vi "ELVIS III v1.0 Read AI.vi"(7 "Scale Constants Array":T1, 8 "error in (no error)":errorcluster, 10 "Channel List":T5, 11 "myRIO Ref In":T3) -> (0 "error out":errorcluster, 2 "dbl Scaled Value List":dbl[](array[numeric]), 3 "myRIO Ref Out":T3)   [LabVIEW 2021]
uses:
  <vilib>/myRIO/Common/Instrument Driver Framework/myRIO v1.0/AI/typedefs/AI Channels List.ctl
  <vilib>/myRIO/Common/Instrument Driver Framework/myRIO v1.0/AI/typedefs/AI Channels Enum.ctl
  <vilib>/myRIO/Common/Instrument Driver Framework/Utilities/typedefs/myRIO v1.0 Reference.ctl
  <vilib>/myRIO/Common/Instrument Driver Framework/Utilities/typedefs/Generic FPGA Reference.ctl
  <vilib>/myRIO/Common/Instrument Driver Framework/Utilities/typedefs/Analog Scaling Constants List.ctl
  <vilib>/myRIO/Common/Instrument Driver Framework/Utilities/typedefs/Analog Scaling Constants.ctl
  <vilib>/myRIO/Common/Instrument Driver Framework/ELVIS III v1.0/AI/typedefs/ELVIS III AI Channels FPGA Reference.ctl
  <vilib>/rvi/errors/niLvFpgaAdjustHostInterfaceError.vi
  <vilib>/rvi/interface/nirviReadWriteControl/nirviReadWriteControl.xnode
  <vilib>/rvi/interface/Simulation/niFpgaSimulationCallBeginRW.vi
  NiFpgaLv.dll
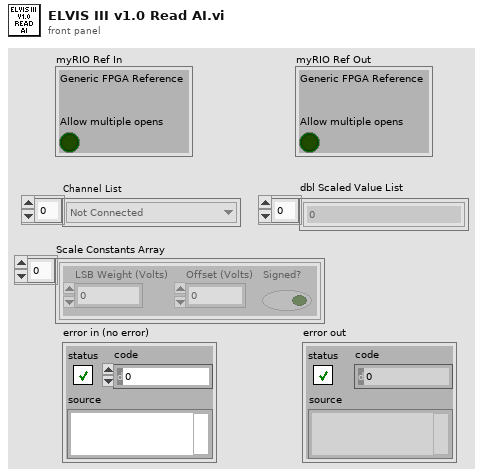
[diagram p1: front panel]
types:
  T1 = typedef "Analog Scaling Constants List.ctl" = T2[]
  T2 = typedef "Analog Scaling Constants.ctl" = cluster{"LSB Weight (Volts)":dbl, "Offset (Volts)":dbl, "Signed?":bool}
  T3 = typedef "myRIO v1.0 Reference.ctl" = cluster{"Generic FPGA Reference":T4, "Allow multiple opens":bool}
  T4 = typedef "Generic FPGA Reference.ctl" = refnum<k20>
  T5 = typedef "AI Channels List.ctl" = T6[]
  T6 = typedef "AI Channels Enum.ctl" = enum16{"Not Connected", "AudioIn/Left", "AudioIn/Right", "C/AI0", "C/AI1", "A/AI0", "A/AI1", "A/AI2", "A/AI3", "A/AI4", "A/AI5", "A/AI6", "A/AI7", "B/AI0", "B/AI1", "B/AI2", "B/AI3", "B/AI4", "B/AI5", "B/AI6", "B/AI7", "AI/AI0", "AI/AI1", "AI/AI2", "AI/AI3", "A/AI0 (DIFF)", "A/AI1 (DIFF)", "A/AI2 (DIFF)", "A/AI3 (DIFF)", "B/AI0 (DIFF)", "B/AI1 (DIFF)", "B/AI2 (DIFF)", "B/AI3 (DIFF)"}
  T7 = typedef "ELVIS III AI Channels FPGA Reference.ctl" = refnum<k20>
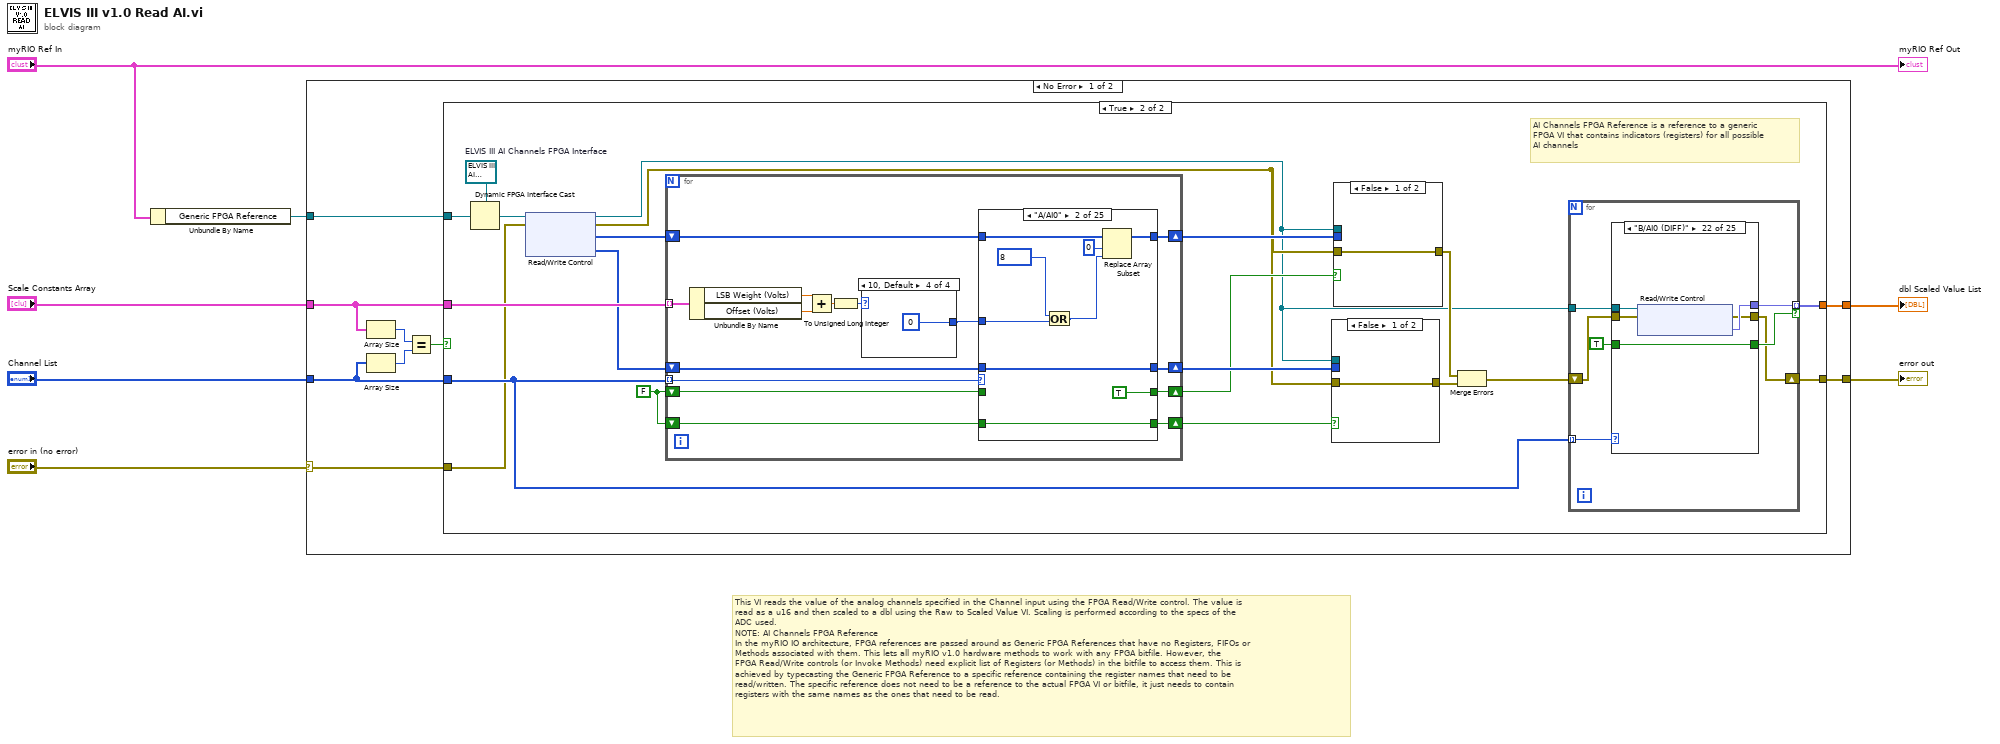
[diagram p0: block diagram]
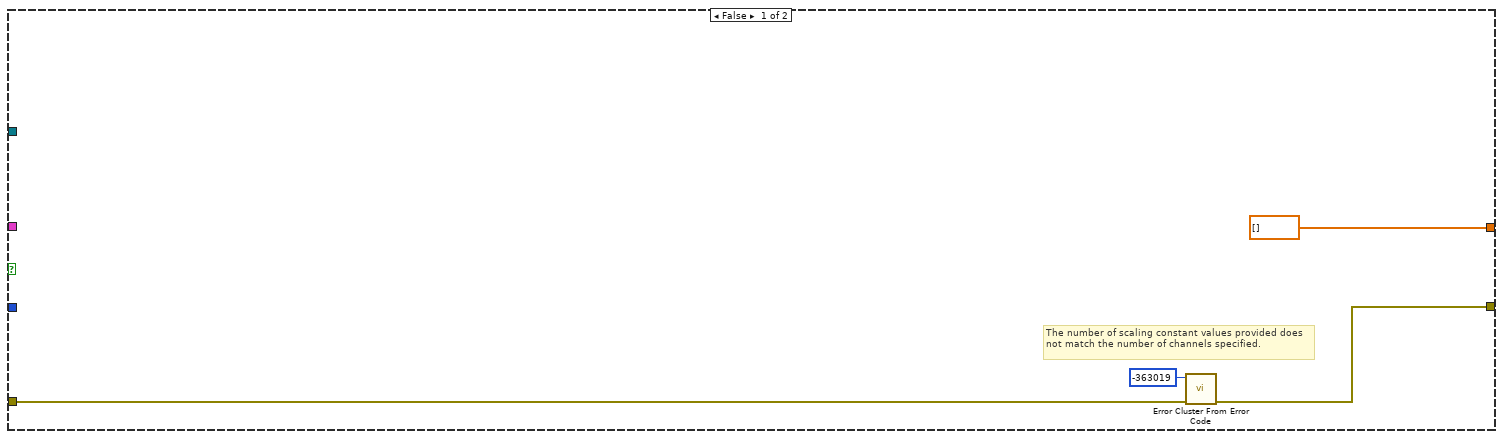
[diagram p2: hidden frame]
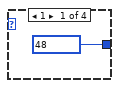
[diagram p3: hidden frame]
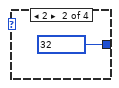
[diagram p4: hidden frame]
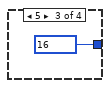
[diagram p5: hidden frame]
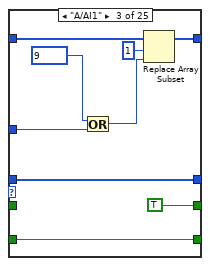
[diagram p7: hidden frame]
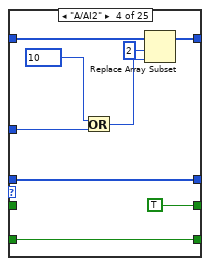
[diagram p8: hidden frame]
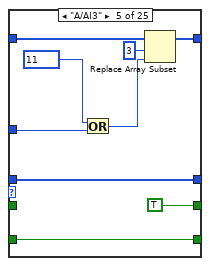
[diagram p9: hidden frame]
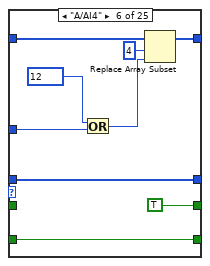
[diagram p10: hidden frame]
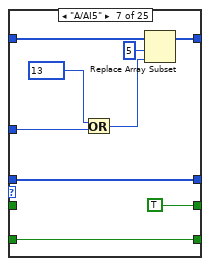
[diagram p11: hidden frame]
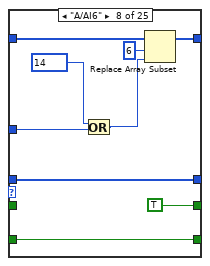
[diagram p12: hidden frame]
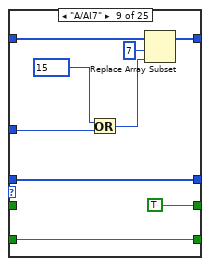
[diagram p13: hidden frame]
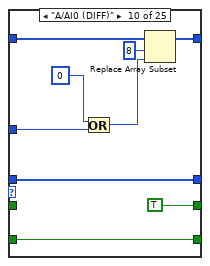
[diagram p14: hidden frame]
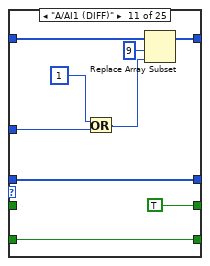
[diagram p15: hidden frame]
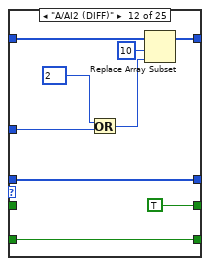
[diagram p16: hidden frame]
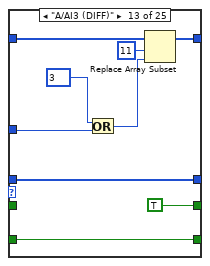
[diagram p17: hidden frame]
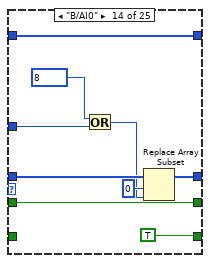
[diagram p18: hidden frame]
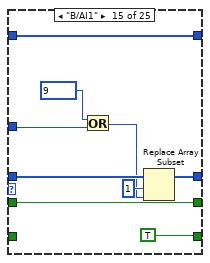
[diagram p19: hidden frame]
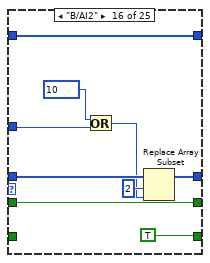
[diagram p20: hidden frame]
diagram:
  # "This VI reads the value of the analog channels specified in the Channel input using the FPGA Read/Write control. The value is \nread as a u16 and then scaled to a dbl using the Raw to Scaled Value VI. Scaling is performed according to the specs of the \nADC used.\nNOTE: AI Channels FPGA Reference\nIn the myRIO IO architecture, FPGA references are passed around as Generic FPGA References that have no Registers, FIFOs or\nMethods associated with them. This lets all myRIO v1.0 hardware methods to work with any FPGA bitfile. However, the \nFPGA Read/Write controls (or Invoke Methods) need explicit list of Registers (or Methods) in the bitfile to access them. This is \nachieved by typecasting the Generic FPGA Reference to a specific reference containing the register names that need to be \nread/written. The specific reference does not need to be a reference to the actual FPGA VI or bitfile, it just needs to contain \nregisters with the same names as the ones that need to be read."
  n1 = Unbundle By Name("myRIO Ref In") -> ("Generic FPGA Reference"=w3:T4)
  n2 = case shown="No Error" "error in (no error)" {
    selector: "error in (no error)" -> [w9 w421]
    tunnel: w3 -> [w16 _]
    tunnel: [w15 w421] -> w7
    tunnel: "Channel List" -> [w13 _]
    tunnel: "Scale Constants Array" -> [w14 _]
    tunnel: [w8 dbl[] []] -> w1
    frame No Error {
      n3 = Array Size(array=w14) -> (size(s)=w12:i32)
      n4 = Array Size(array=w13) -> (size(s)=w11:i32)
      n5 = Equal?(x=w12, y=w11) -> (x = y?=w10:bool)
      n6 = case shown="True" w10 {
        tunnel: w16 -> [_ w39]
        tunnel: [w20 w38] -> w15
        tunnel: w13 -> [_ w31]
        tunnel: w14 -> [_ w30]
        tunnel: w9 -> [w17 w25]
        tunnel: [dbl[] [] w35] -> w8
        frame False {
          # "The number of scaling constant values provided does not match the number of channels specified."
          n7 = call <vilib>:"Error Cluster From Error Code.vi"("error in (no error)"=w17, "error code (0)"=-363019) -> ("error out"=w20:errorcluster)  [unwired: 7 in]
        }
        frame True {
          w33 = FALSE
          w40 = T7 refnum  # ELVIS III AI Channels FPGA Interface
          # "AI Channels FPGA Reference is a reference to a generic FPGA VI that contains indicators (registers) for all possible AI channels"
          n8 = Dynamic FPGA Interface Cast(Session In=w40, Type=w39) -> (Session Out=w34:T7)
          n9 = xnode "Read/Write Control"("FPGA VI Reference In"=w34, "error in"=w25) -> ("FPGA VI Reference Out"=w21:T7, "error out"=w23:errorcluster, "AI.A.CNFG"=w32:u8[], "AI.B.CNFG"=w24:u8[])
          n10 = for {
            tunnel: w30 -> [w42] mode=indexing
            shift-right: [w54] -> w29
            shift-left: w32 -> [w55]
            shift-right: [w52] -> w28
            shift-left: w24 -> [w53]
            shift-right: [w50] -> w27
            shift-left: w33 -> [w51]
            shift-right: [w48] -> w26
            shift-left: w33 -> [w49]
            tunnel: w31 -> [w47] mode=indexing
            n11 = Unbundle By Name(w42) -> ("LSB Weight (Volts)"=w45:dbl, "Offset (Volts)"=w46:dbl)
            n12 = Add(x=w45, y=w46) -> (x+y=w44:dbl)
            n13 = To Unsigned Long Integer(number=w44) -> (unsigned 32bit integer=w43:u32)
            n14 = case shown="10, Default" w43 {
              tunnel: [u8 48 u8 32 u8 16 u8 0] -> w41
              frame 1 {
              }
              frame 2 {
              }
              frame 5 {
              }
              frame 10, Default {
              }
            }
            n15 = case shown="\"A/AI0\"" w47 {
              tunnel: w55 -> [w62 w71 w79 w89 w98 w106 w115 w124 w133 w142 w151 w160 w169 w180 w189 w198 w207 w216 w225 w234 w243 w252 w261 w270 w279]
              tunnel: [w62 w70 w80 w88 w97 w107 w116 w125 w134 w143 w152 w161 w170 w180 w189 w198 w207 w216 w225 w234 w243 w252 w261 w270 w279] -> w54
              tunnel: w53 -> [w63 w69 w78 w87 w96 w105 w114 w123 w132 w141 w150 w159 w168 w177 w186 w195 w204 w213 w222 w231 w240 w249 w258 w267 w276]
              tunnel: [w63 w69 w78 w87 w96 w105 w114 w123 w132 w141 w150 w159 w168 w178 w187 w196 w205 w214 w223 w232 w241 w250 w259 w268 w277] -> w52
              tunnel: w51 -> [w61 _ _ _ _ _ _ _ _ _ _ _ _ w176 w185 w194 w203 w212 w221 w230 w239 w248 w257 w266 w275]
              tunnel: [w61 TRUE TRUE TRUE TRUE TRUE TRUE TRUE TRUE TRUE TRUE TRUE TRUE w176 w185 w194 w203 w212 w221 w230 w239 w248 w257 w266 w275] -> w50
              tunnel: w49 -> [w60 w67 w76 w85 w94 w103 w112 w121 w130 w139 w148 w157 w166 _ _ _ _ _ _ _ _ _ _ _ _]
              tunnel: [w60 w67 w76 w85 w94 w103 w112 w121 w130 w139 w148 w157 w166 TRUE TRUE TRUE TRUE TRUE TRUE TRUE TRUE TRUE TRUE TRUE TRUE] -> w48
              tunnel: w41 -> [_ w64 w73 w82 w91 w100 w109 w118 w127 w136 w145 w154 w163 w172 w181 w190 w199 w208 w217 w226 w235 w244 w253 w262 w271]
              frame Default {
              }
              frame "A/AI0" {
                n16 = Or(x=u8 8, y=w64) -> (x .or. y?=w65:u8)
                n17 = Replace Array Subset(array=w71, new element=w65, index=0) -> (w70:u8[])
              }
              frame "A/AI1" {
                n18 = Or(x=u8 9, y=w73) -> (x .or. y?=w74:u8)
                n19 = Replace Array Subset(array=w79, new element=w74, index=1) -> (w80:u8[])
              }
              frame "A/AI2" {
                n20 = Or(x=u8 10, y=w82) -> (x .or. y?=w83:u8)
                n21 = Replace Array Subset(array=w89, new element=w83, index=2) -> (w88:u8[])
              }
              frame "A/AI3" {
                n22 = Or(x=u8 11, y=w91) -> (x .or. y?=w92:u8)
                n23 = Replace Array Subset(array=w98, new element=w92, index=3) -> (w97:u8[])
              }
              frame "A/AI4" {
                n24 = Or(x=u8 12, y=w100) -> (x .or. y?=w101:u8)
                n25 = Replace Array Subset(array=w106, new element=w101, index=4) -> (w107:u8[])
              }
              frame "A/AI5" {
                n26 = Or(x=u8 13, y=w109) -> (x .or. y?=w110:u8)
                n27 = Replace Array Subset(array=w115, new element=w110, index=5) -> (w116:u8[])
              }
              frame "A/AI6" {
                n28 = Or(x=u8 14, y=w118) -> (x .or. y?=w119:u8)
                n29 = Replace Array Subset(array=w124, new element=w119, index=6) -> (w125:u8[])
              }
              frame "A/AI7" {
                n30 = Or(x=u8 15, y=w127) -> (x .or. y?=w128:u8)
                n31 = Replace Array Subset(array=w133, new element=w128, index=7) -> (w134:u8[])
              }
              frame "A/AI0 (DIFF)" {
                n32 = Or(x=u8 0, y=w136) -> (x .or. y?=w137:u8)
                n33 = Replace Array Subset(array=w142, new element=w137, index=8) -> (w143:u8[])
              }
              frame "A/AI1 (DIFF)" {
                n34 = Or(x=u8 1, y=w145) -> (x .or. y?=w146:u8)
                n35 = Replace Array Subset(array=w151, new element=w146, index=9) -> (w152:u8[])
              }
              frame "A/AI2 (DIFF)" {
                n36 = Or(x=u8 2, y=w154) -> (x .or. y?=w155:u8)
                n37 = Replace Array Subset(array=w160, new element=w155, index=10) -> (w161:u8[])
              }
              frame "A/AI3 (DIFF)" {
                n38 = Or(x=u8 3, y=w163) -> (x .or. y?=w164:u8)
                n39 = Replace Array Subset(array=w169, new element=w164, index=11) -> (w170:u8[])
              }
              frame "B/AI0" {
                n40 = Or(x=u8 8, y=w172) -> (x .or. y?=w173:u8)
                n41 = Replace Array Subset(array=w177, new element=w173, index=0) -> (w178:u8[])
              }
              frame "B/AI1" {
                n42 = Or(x=u8 9, y=w181) -> (x .or. y?=w183:u8)
                n43 = Replace Array Subset(array=w186, new element=w183, index=1) -> (w187:u8[])
              }
              frame "B/AI2" {
                n44 = Or(x=u8 10, y=w190) -> (x .or. y?=w192:u8)
                n45 = Replace Array Subset(array=w195, new element=w192, index=2) -> (w196:u8[])
              }
              frame "B/AI3" {
                n46 = Or(x=u8 11, y=w199) -> (x .or. y?=w200:u8)
                n47 = Replace Array Subset(array=w204, new element=w200, index=3) -> (w205:u8[])
              }
              frame "B/AI4" {
                n48 = Or(x=u8 12, y=w208) -> (x .or. y?=w209:u8)
                n49 = Replace Array Subset(array=w213, new element=w209, index=4) -> (w214:u8[])
              }
              frame "B/AI5" {
                n50 = Or(x=u8 13, y=w217) -> (x .or. y?=w218:u8)
                n51 = Replace Array Subset(array=w222, new element=w218, index=5) -> (w223:u8[])
              }
              frame "B/AI6" {
                n52 = Or(x=u8 14, y=w226) -> (x .or. y?=w228:u8)
                n53 = Replace Array Subset(array=w231, new element=w228, index=6) -> (w232:u8[])
              }
              frame "B/AI7" {
                n54 = Or(x=u8 15, y=w235) -> (x .or. y?=w237:u8)
                n55 = Replace Array Subset(array=w240, new element=w237, index=7) -> (w241:u8[])
              }
              frame "B/AI0 (DIFF)" {
                n56 = Or(x=u8 0, y=w244) -> (x .or. y?=w245:u8)
                n57 = Replace Array Subset(array=w249, new element=w245, index=8) -> (w250:u8[])
              }
              frame "B/AI1 (DIFF)" {
                n58 = Or(x=u8 1, y=w253) -> (x .or. y?=w255:u8)
                n59 = Replace Array Subset(array=w258, new element=w255, index=9) -> (w259:u8[])
              }
              frame "B/AI2 (DIFF)" {
                n60 = Or(x=u8 2, y=w262) -> (x .or. y?=w264:u8)
                n61 = Replace Array Subset(array=w267, new element=w264, index=10) -> (w268:u8[])
              }
              frame "B/AI3 (DIFF)" {
                n62 = Or(x=u8 3, y=w271) -> (x .or. y?=w273:u8)
                n63 = Replace Array Subset(array=w276, new element=w273, index=11) -> (w277:u8[])
              }
            }
          }
          n64 = case shown="False" w26 {
            tunnel: w23 -> [w280 w282]
            tunnel: w28 -> [_ w283]
            tunnel: [w280 w281] -> w36
            tunnel: w21 -> [_ w284]
            frame False {
            }
            frame True {
              n65 = call <vilib>:"ELVIS III v1.0 AI Read Bank B.vi"("error in (no error)"=w282, "AI.B.CNFG"=w283, "Refnum in"=w284) -> ("error out"=w281:errorcluster)  [unwired: 8 in]
            }
          }
          n66 = case shown="False" w27 {
            tunnel: w21 -> [_ w289]
            tunnel: w29 -> [_ w287]
            tunnel: w23 -> [w285 w288]
            tunnel: [w285 w286] -> w37
            frame False {
            }
            frame True {
              n67 = call <vilib>:"ELVIS III v1.0 AI Read Bank A.vi"("error in (no error)"=w288, "AI.A.CNFG"=w287, "Refnum in"=w289) -> ("error out"=w286:errorcluster)  [unwired: 8 in]
            }
          }
          n68 = Merge Errors(w37, w36) -> (w22:errorcluster)
          n69 = for {
            shift-right: [w290] -> w38
            shift-left: w22 -> [w291]
            tunnel: w31 -> [w296] mode=indexing
            tunnel: [w295] -> w35 mode=indexing if=w294
            tunnel: w21 -> [w292]
            n70 = case shown="\"B/AI0 (DIFF)\"" w296 {
              tunnel: [fxp<+/-,26,5> 0.0 ("Analog In (1 Sample)") w302 w307 w312 w317 w322 w327 w332 w337 w342 w347 w352 w357 w362 w367 w372 w377 w382 w387 w392 w397 w402 w407 w412 w417] -> w295
              tunnel: [FALSE w304 w309 w314 w319 w324 w329 w334 w339 w344 w349 w354 w359 w364 w369 w374 w379 w384 w389 w394 w399 w404 w409 w414 w419] -> w294
              tunnel: TRUE -> [_ w304 w309 w314 w319 w324 w329 w334 w339 w344 w349 w354 w359 w364 w369 w374 w379 w384 w389 w394 w399 w404 w409 w414 w419]
              tunnel: w292 -> [_ w303 w308 w313 w318 w323 w328 w333 w338 w343 w348 w353 w358 w363 w368 w373 w378 w383 w388 w393 w398 w403 w408 w413 w418]
              tunnel: w291 -> [w297 w301 w306 w311 w316 w321 w326 w331 w336 w341 w346 w351 w356 w361 w366 w371 w376 w381 w386 w391 w396 w401 w406 w411 w416]
              tunnel: [w297 w300 w305 w310 w315 w320 w325 w330 w335 w340 w345 w350 w355 w360 w365 w370 w375 w380 w385 w390 w395 w400 w405 w410 w415] -> w290
              frame Default {
              }
              frame "A/AI0" {
                n71 = xnode "Read/Write Control"("FPGA VI Reference In"=w303, "error in"=w301) -> ("error out"=w300:errorcluster, "AI.A_0.VAL"=w302:fxp<+/-,26,5>)  [unwired: 1 out]
              }
              frame "A/AI1" {
                n72 = xnode "Read/Write Control"("FPGA VI Reference In"=w308, "error in"=w306) -> ("error out"=w305:errorcluster, "AI.A_1.VAL"=w307:fxp<+/-,26,5>)  [unwired: 1 out]
              }
              frame "A/AI2" {
                n73 = xnode "Read/Write Control"("FPGA VI Reference In"=w313, "error in"=w311) -> ("error out"=w310:errorcluster, "AI.A_2.VAL"=w312:fxp<+/-,26,5>)  [unwired: 1 out]
              }
              frame "A/AI3" {
                n74 = xnode "Read/Write Control"("FPGA VI Reference In"=w318, "error in"=w316) -> ("error out"=w315:errorcluster, "AI.A_3.VAL"=w317:fxp<+/-,26,5>)  [unwired: 1 out]
              }
              frame "A/AI4" {
                n75 = xnode "Read/Write Control"("FPGA VI Reference In"=w323, "error in"=w321) -> ("error out"=w320:errorcluster, "AI.A_4.VAL"=w322:fxp<+/-,26,5>)  [unwired: 1 out]
              }
              frame "A/AI5" {
                n76 = xnode "Read/Write Control"("FPGA VI Reference In"=w328, "error in"=w326) -> ("error out"=w325:errorcluster, "AI.A_5.VAL"=w327:fxp<+/-,26,5>)  [unwired: 1 out]
              }
              frame "A/AI6" {
                n77 = xnode "Read/Write Control"("FPGA VI Reference In"=w333, "error in"=w331) -> ("error out"=w330:errorcluster, "AI.A_6.VAL"=w332:fxp<+/-,26,5>)  [unwired: 1 out]
              }
              frame "A/AI7" {
                n78 = xnode "Read/Write Control"("FPGA VI Reference In"=w338, "error in"=w336) -> ("error out"=w335:errorcluster, "AI.A_7.VAL"=w337:fxp<+/-,26,5>)  [unwired: 1 out]
              }
              frame "A/AI0 (DIFF)" {
                n79 = xnode "Read/Write Control"("FPGA VI Reference In"=w343, "error in"=w341) -> ("error out"=w340:errorcluster, "AI.DIFF_A_0.VAL"=w342:fxp<+/-,26,5>)  [unwired: 1 out]
              }
              frame "A/AI1 (DIFF)" {
                n80 = xnode "Read/Write Control"("FPGA VI Reference In"=w348, "error in"=w346) -> ("error out"=w345:errorcluster, "AI.DIFF_A_1.VAL"=w347:fxp<+/-,26,5>)  [unwired: 1 out]
              }
              frame "A/AI2 (DIFF)" {
                n81 = xnode "Read/Write Control"("FPGA VI Reference In"=w353, "error in"=w351) -> ("error out"=w350:errorcluster, "AI.DIFF_A_2.VAL"=w352:fxp<+/-,26,5>)  [unwired: 1 out]
              }
              frame "A/AI3 (DIFF)" {
                n82 = xnode "Read/Write Control"("FPGA VI Reference In"=w358, "error in"=w356) -> ("error out"=w355:errorcluster, "AI.DIFF_A_3.VAL"=w357:fxp<+/-,26,5>)  [unwired: 1 out]
              }
              frame "B/AI0" {
                n83 = xnode "Read/Write Control"("FPGA VI Reference In"=w363, "error in"=w361) -> ("error out"=w360:errorcluster, "AI.B_0.VAL"=w362:fxp<+/-,26,5>)  [unwired: 1 out]
              }
              frame "B/AI1" {
                n84 = xnode "Read/Write Control"("FPGA VI Reference In"=w368, "error in"=w366) -> ("error out"=w365:errorcluster, "AI.B_1.VAL"=w367:fxp<+/-,26,5>)  [unwired: 1 out]
              }
              frame "B/AI2" {
                n85 = xnode "Read/Write Control"("FPGA VI Reference In"=w373, "error in"=w371) -> ("error out"=w370:errorcluster, "AI.B_2.VAL"=w372:fxp<+/-,26,5>)  [unwired: 1 out]
              }
              frame "B/AI3" {
                n86 = xnode "Read/Write Control"("FPGA VI Reference In"=w378, "error in"=w376) -> ("error out"=w375:errorcluster, "AI.B_3.VAL"=w377:fxp<+/-,26,5>)  [unwired: 1 out]
              }
              frame "B/AI4" {
                n87 = xnode "Read/Write Control"("FPGA VI Reference In"=w383, "error in"=w381) -> ("error out"=w380:errorcluster, "AI.B_4.VAL"=w382:fxp<+/-,26,5>)  [unwired: 1 out]
              }
              frame "B/AI5" {
                n88 = xnode "Read/Write Control"("FPGA VI Reference In"=w388, "error in"=w386) -> ("error out"=w385:errorcluster, "AI.B_5.VAL"=w387:fxp<+/-,26,5>)  [unwired: 1 out]
              }
              frame "B/AI6" {
                n89 = xnode "Read/Write Control"("FPGA VI Reference In"=w393, "error in"=w391) -> ("error out"=w390:errorcluster, "AI.B_6.VAL"=w392:fxp<+/-,26,5>)  [unwired: 1 out]
              }
              frame "B/AI7" {
                n90 = xnode "Read/Write Control"("FPGA VI Reference In"=w398, "error in"=w396) -> ("error out"=w395:errorcluster, "AI.B_7.VAL"=w397:fxp<+/-,26,5>)  [unwired: 1 out]
              }
              frame "B/AI0 (DIFF)" {
                n91 = xnode "Read/Write Control"("FPGA VI Reference In"=w403, "error in"=w401) -> ("error out"=w400:errorcluster, "AI.DIFF_B_0.VAL"=w402:fxp<+/-,26,5>)  [unwired: 1 out]
              }
              frame "B/AI1 (DIFF)" {
                n92 = xnode "Read/Write Control"("FPGA VI Reference In"=w408, "error in"=w406) -> ("error out"=w405:errorcluster, "AI.DIFF_B_1.VAL"=w407:fxp<+/-,26,5>)  [unwired: 1 out]
              }
              frame "B/AI2 (DIFF)" {
                n93 = xnode "Read/Write Control"("FPGA VI Reference In"=w413, "error in"=w411) -> ("error out"=w410:errorcluster, "AI.DIFF_B_2.VAL"=w412:fxp<+/-,26,5>)  [unwired: 1 out]
              }
              frame "B/AI3 (DIFF)" {
                n94 = xnode "Read/Write Control"("FPGA VI Reference In"=w418, "error in"=w416) -> ("error out"=w415:errorcluster, "AI.DIFF_B_3.VAL"=w417:fxp<+/-,26,5>)  [unwired: 1 out]
              }
            }
          }
        }
      }
    }
    frame Error {
      # "There is an incoming error so there it nothing to do."
    }
  }
  "error out" <- w7
  "dbl Scaled Value List" <- w1
  "myRIO Ref Out" <- "myRIO Ref In"
